vi "Initialize.vi"(8 "error in (no error)":errorcluster, 10 "Device in":refnum<class "Device.lvclass">, 11 "IP Connection in":refnum<class "IP Connection.lvclass">) -> (0 "error out":errorcluster, 2 "Device out":refnum<class "Device.lvclass">, 3 "IP Connection out":refnum<class "IP Connection.lvclass">)   [LabVIEW 2011, in "Tinkerforge.lvlib" / "Device.lvclass"]
doc: "This VI initializes the device object with data from the friendly IP connection class."
uses:
  Device.lvclass
  IP Connection/IP Connection.lvclass
  Device.lvclass/Device.ctl
  IP Connection/Properties/Read Synchronization Stuff.vi
  IP Connection/Properties/Read Timeout.vi
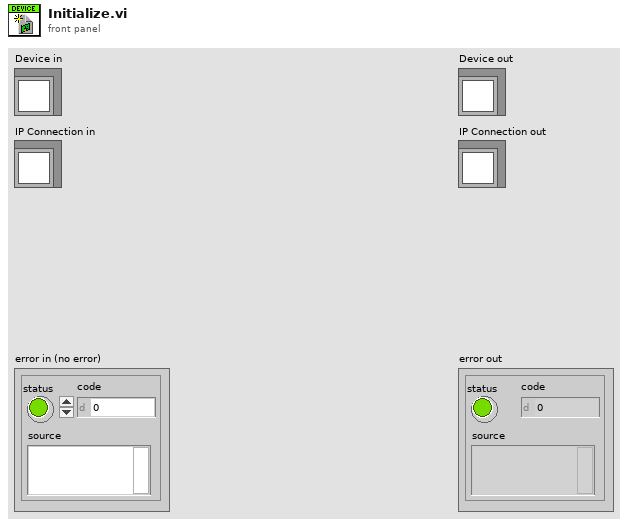
[diagram p1: front panel]
types:
  T1 = typedef "Tinkerforge.lvlib/IP Connection.lvclass/Sync Stuff.ctl" = cluster{"Write":refnum<queue>, "pending Writes":refnum<queue>, "Answer":refnum<user-event>, "Enumerate CB":refnum<user-event>, "Stack":refnum<queue>, "Shutdown":refnum<notifier>}
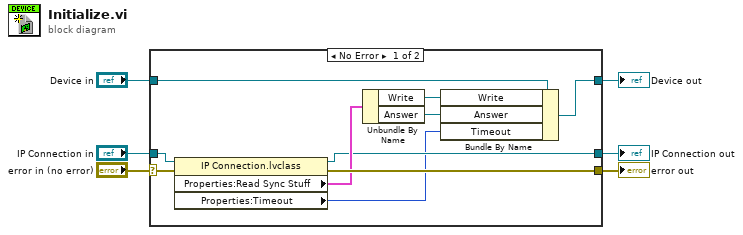
[diagram p0: block diagram]
diagram:
  n1 = case shown="No Error" "error in (no error)" {
    selector: "error in (no error)" -> [w15 w19]
    tunnel: [w14 w19] -> w5
    tunnel: [w9 w18] -> w3
    tunnel: "Device in" -> [w10 w18]
    tunnel: "IP Connection in" -> [w16 w17]
    tunnel: [w8 w17] -> w1
    frame No Error {
      n2 = property class="IP Connection.lvclass"(reference=w16, error in=w15) -> (reference out=w8:refnum<class "IP Connection.lvclass">, error out=w14:errorcluster, "Properties:Read Sync Stuff"=w13:T1, "Properties:Timeout"=w7:i32)
      n3 = Unbundle By Name(w13) -> ("Write"=w12:refnum<queue>, "Answer"=w11:refnum<user-event>)
      n4 = Bundle By Name(cluster=w10, "Write"=w12, "Answer"=w11, "Timeout"=w7) -> (w9:refnum<class "Device.lvclass">)
    }
    frame Error {
    }
  }
  "error out" <- w5
  "Device out" <- w3
  "IP Connection out" <- w1
